vi "main.vi"() -> ()   [LabVIEW 2023]
uses:
  <vilib>/vision/Image Controls.llb/IMAQ Image.ctl
  <vilib>/vision/Shape Detection.llb/ShapeDetectionMatchOptions.ctl
  <vilib>/vision/Pattern Matching.llb/IMAQ Match Range Setting.ctl
  <vilib>/vision/NI_Vision_Development_Module.lvlib
panel:
  out "Triangles":i32
  out "String":string
  out "Rectangles":i32
  out "Circles":i32
  out "Obraz":T1(plugin-control)
  in  "Output Path":path
  in  "Input Path":path=path "C:/Users/kacpe/Desktop/OSP/testp.png"
  in  "Refresh Button":bool
  in  "Process Stop Button":bool
  in  "Save As Button":bool
  in  "Open Button":bool
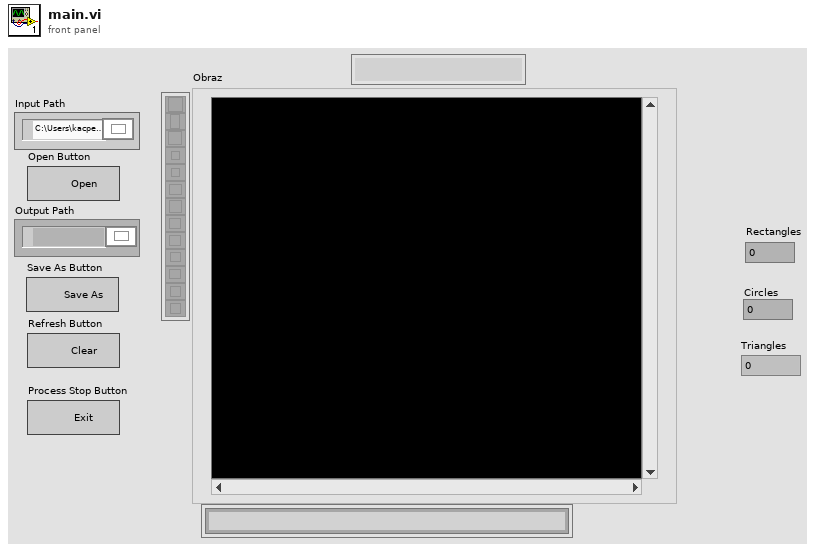
[diagram p1: front panel]
types:
  T1 = typedef "IMAQ Image.ctl" = refnum<image>
  T2 = enum32{"Invalid", "Standard", "Closed", "Hidden", "Minimized", "Maximized"}
  T3 = enum32{"invalid app kind", "Development System", "Run Time System", "Student Edition", "Embedded LabVIEW", "Evaluation", "Custom"}
  T4 = cluster{"Position":cluster{"x":sgl, "y":sgl}, "Angle":sgl, "Scale":sgl, "Score":sgl, "Bounding Box":cluster{"x":sgl, "y":sgl}[]}[]
  T5 = cluster{"Corners":cluster{"X":sgl, "Y":sgl}[], "Angle":dbl, "Width":dbl, "Height":dbl, "Score":dbl}[]
  T6 = cluster{"Position":cluster{"X":sgl, "Y":sgl}, "Radius":dbl, "Score":dbl}[]
  T7 = cluster{"Left":i32, "Top":i32, "Right":i32, "Bottom":i32}
  T8 = cluster{"Min Width":dbl, "Max Width":dbl, "Min Height":dbl, "Max Height":dbl}
  T9 = cluster{"Core":cluster{"Current VI Reference":refnum<vi>, "Close Panel on Exit?":bool}, "Obraz":T1, enum16{"null", "kwadrat", "kolo", "trojkat"}, "Rectangles 2":cluster{"Corners":cluster{"X":sgl, "Y":sgl}[], "Angle":dbl, "Width":dbl, "Height":dbl, "Score":dbl}[], "Circles":cluster{"Position":cluster{"X":sgl, "Y":sgl}, "Radius":dbl, "Score":dbl}[], "Matches (pixel)":cluster{"Position":cluster{"x":sgl, "y":sgl}, "Angle":sgl, "Scale":sgl, "Score":sgl, "Bounding Box":cluster{"x":sgl, "y":sgl}[]}[], "Znak":string}
  T10 = cluster{"Current VI Reference":refnum<vi>, "Close Panel on Exit?":bool}
  T11 = cluster{"Position":cluster{"x":sgl, "y":sgl}, "Angle":sgl, "Scale":sgl, "Score":sgl, "Bounding Box":cluster{"x":sgl, "y":sgl}[]}
  T12 = typedef "ShapeDetectionMatchOptions.ctl" = cluster{"Rotation":bool, "Scale":bool, "Occlusion":bool, "Range Settings":T13[]}
  T13 = typedef "IMAQ Match Range Setting.ctl" = cluster{"Match Constraints":u32, "Min":dbl, "Max":dbl}
  T14 = typedef "Image Type" = u32
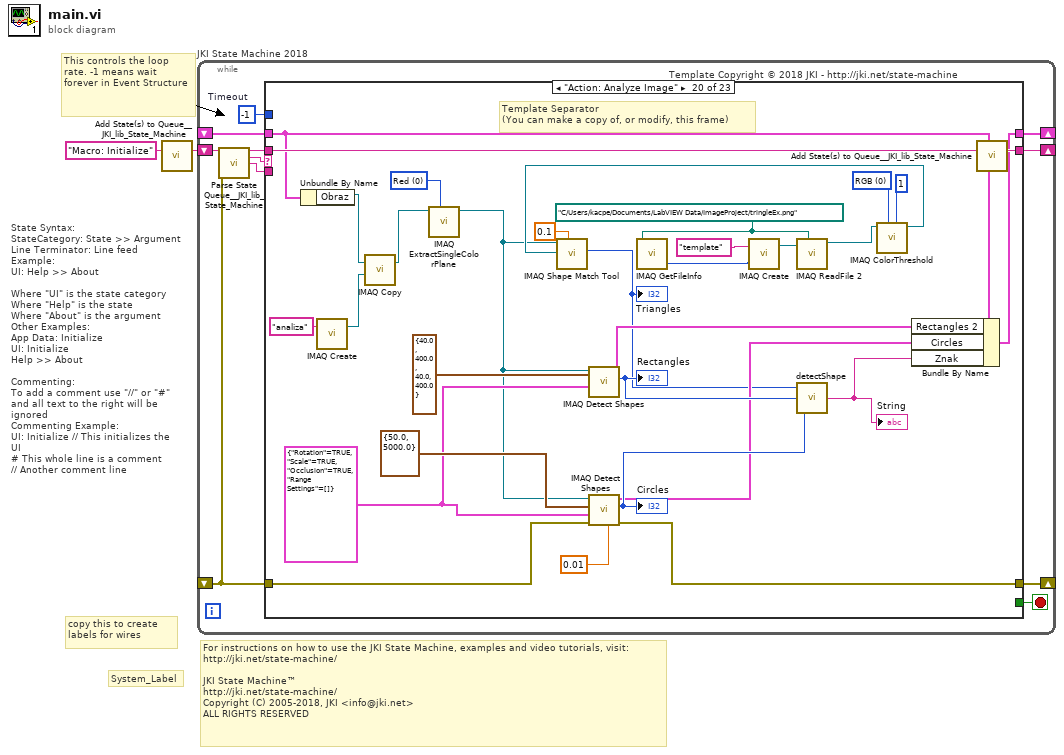
[diagram p0: block diagram]
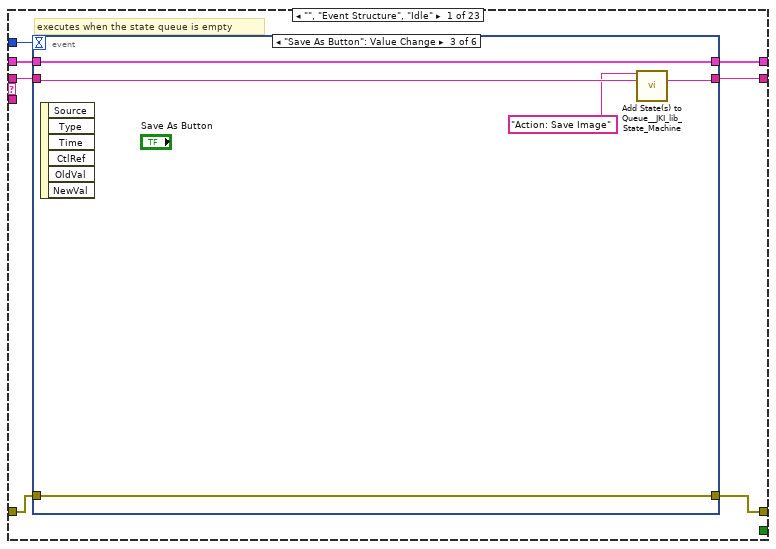
[diagram p2: hidden frame]
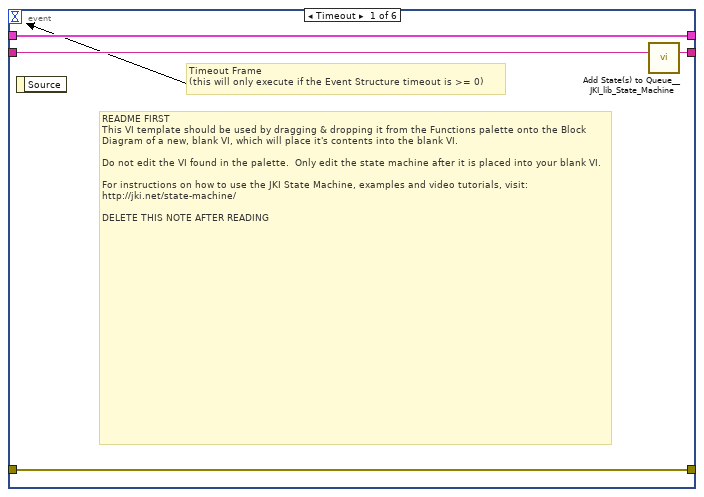
[diagram p3: hidden frame]
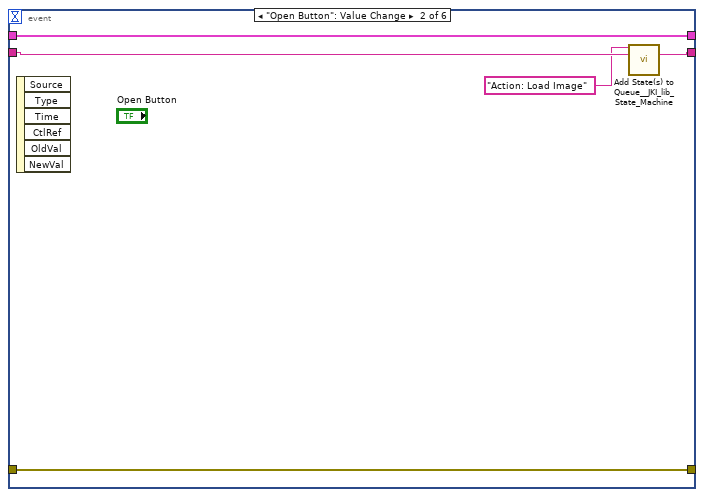
[diagram p4: hidden frame]
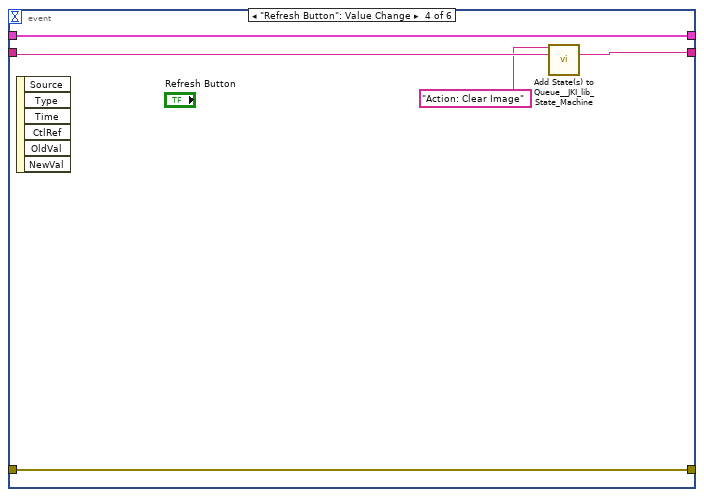
[diagram p5: hidden frame]
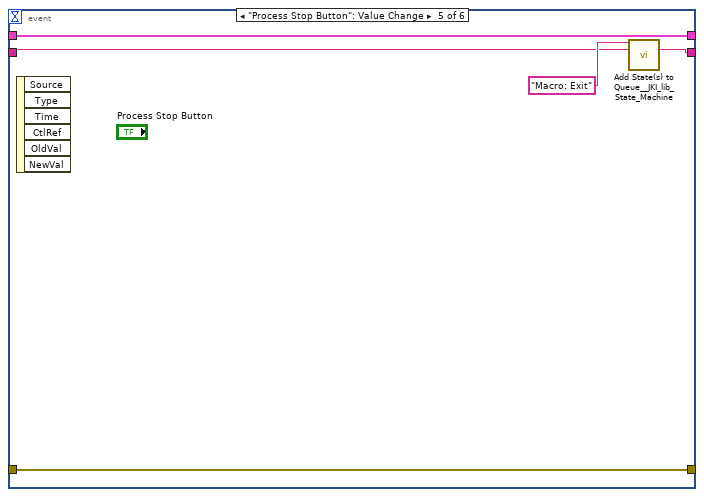
[diagram p6: hidden frame]
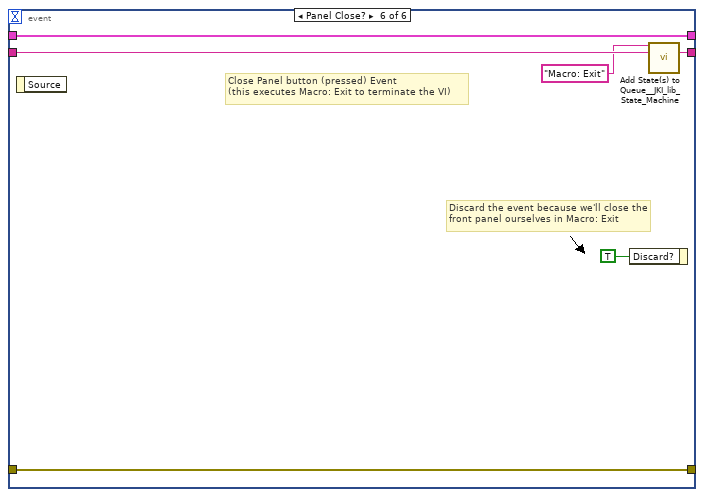
[diagram p7: hidden frame]
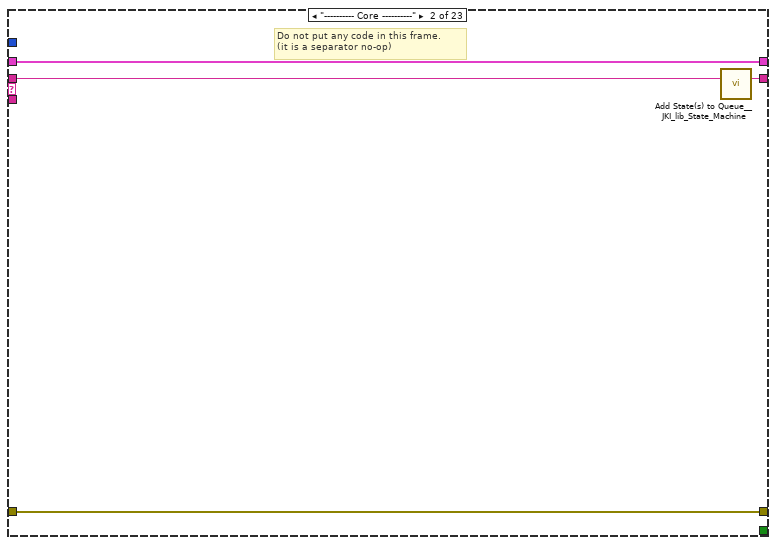
[diagram p8: hidden frame]
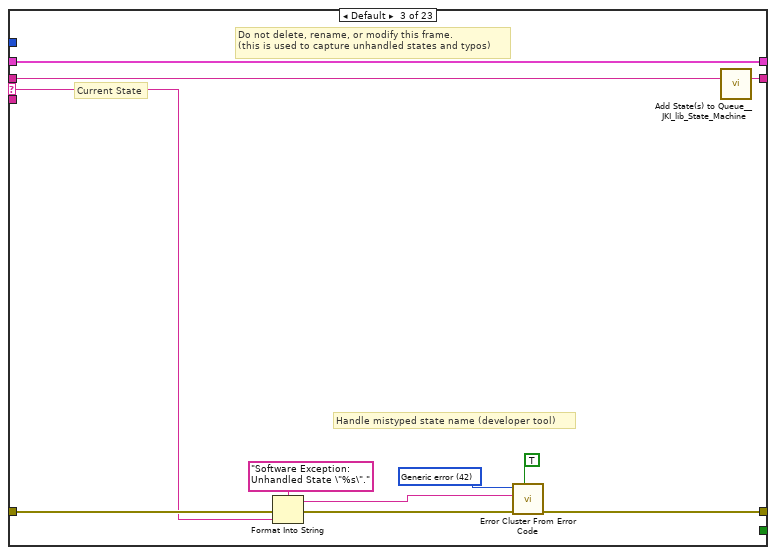
[diagram p9: hidden frame]
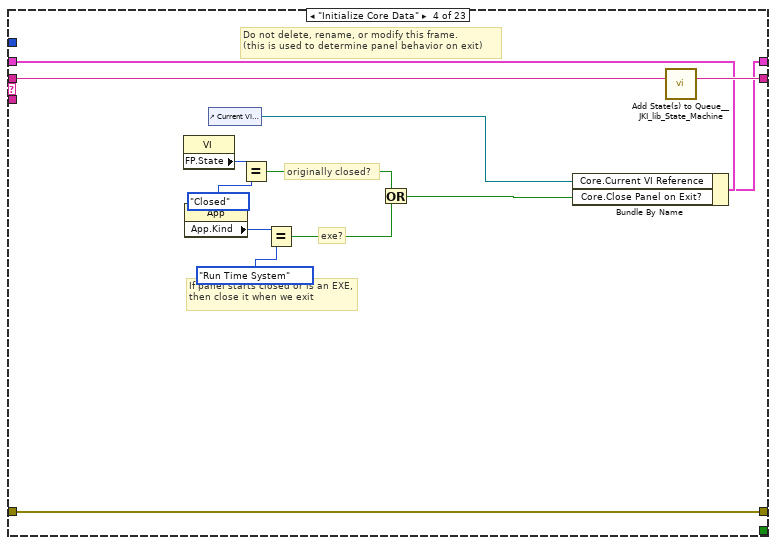
[diagram p10: hidden frame]
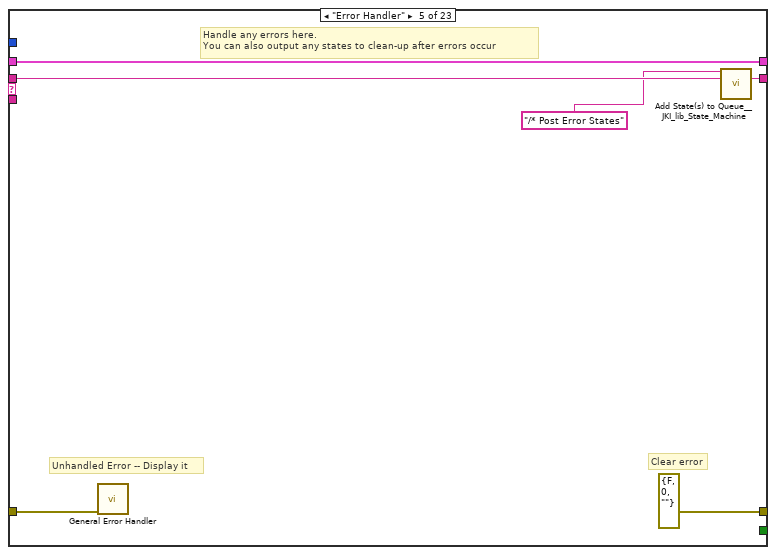
[diagram p11: hidden frame]
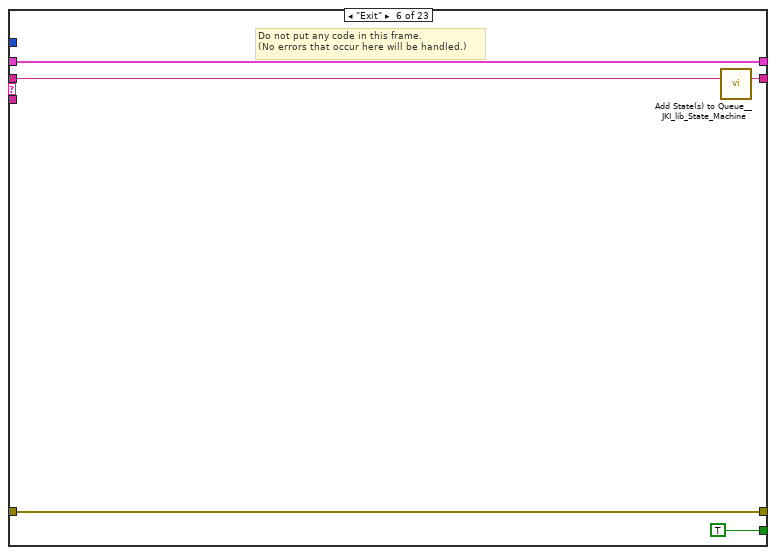
[diagram p12: hidden frame]
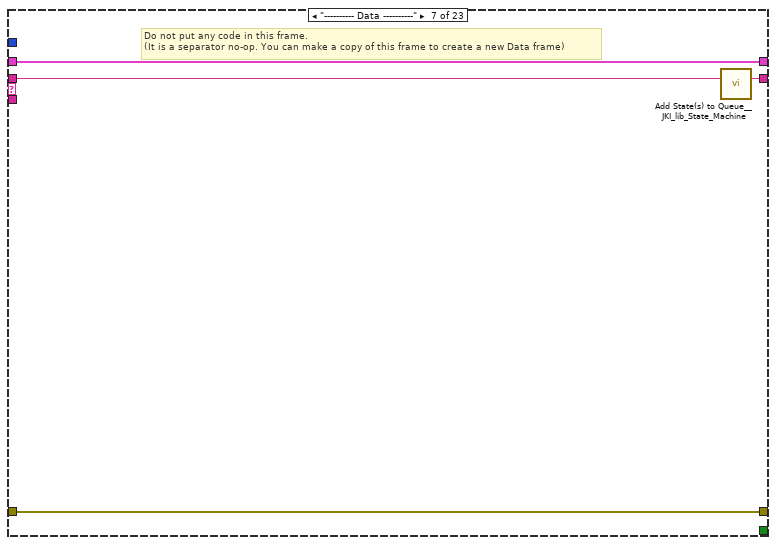
[diagram p13: hidden frame]
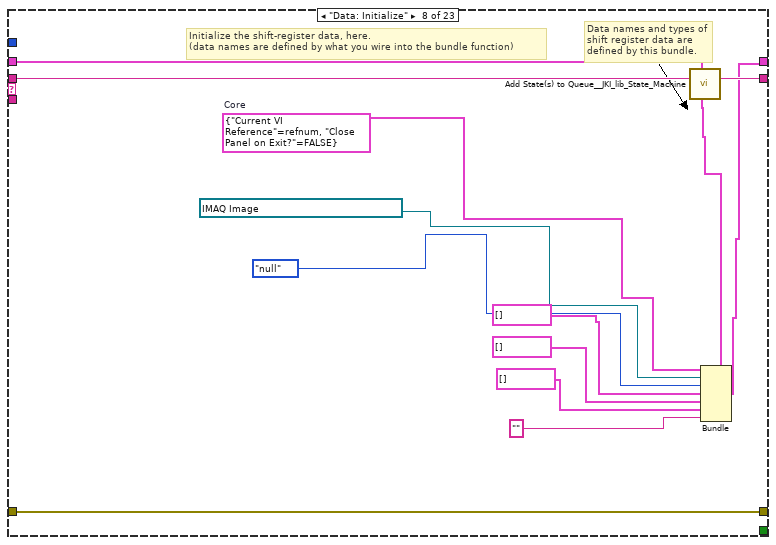
[diagram p14: hidden frame]
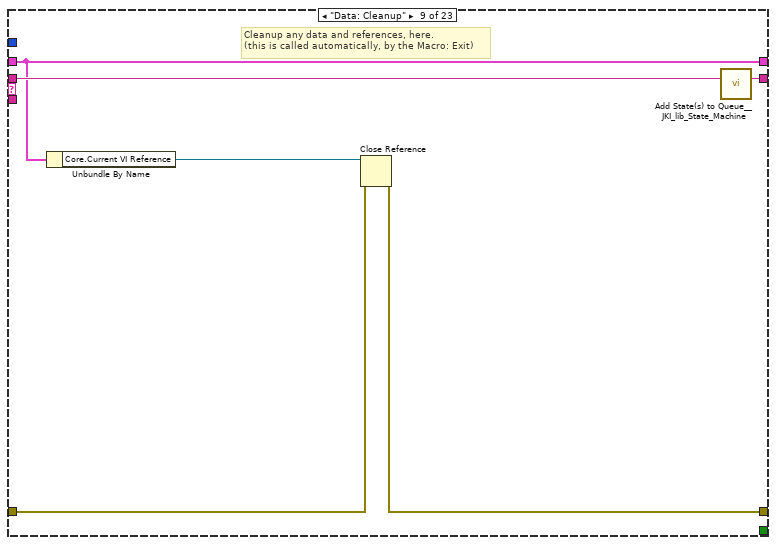
[diagram p15: hidden frame]
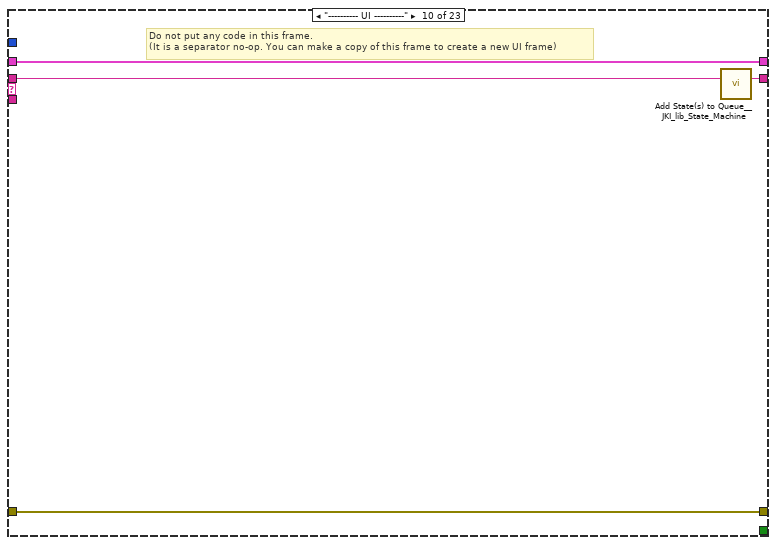
[diagram p16: hidden frame]
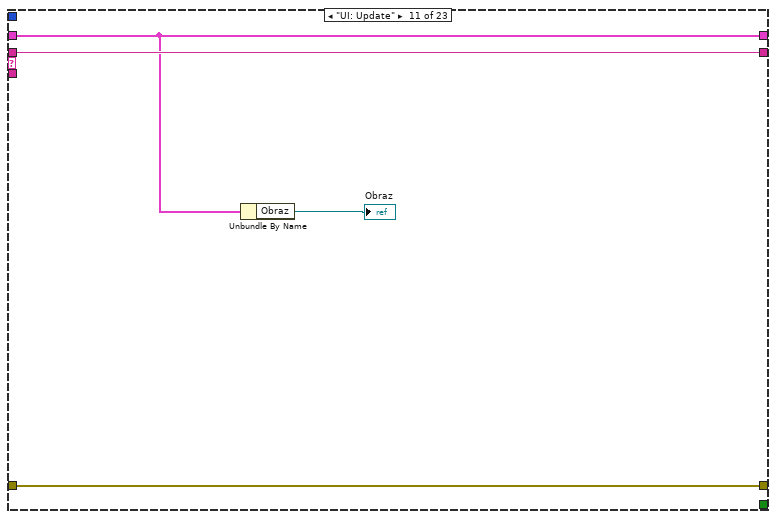
[diagram p17: hidden frame]
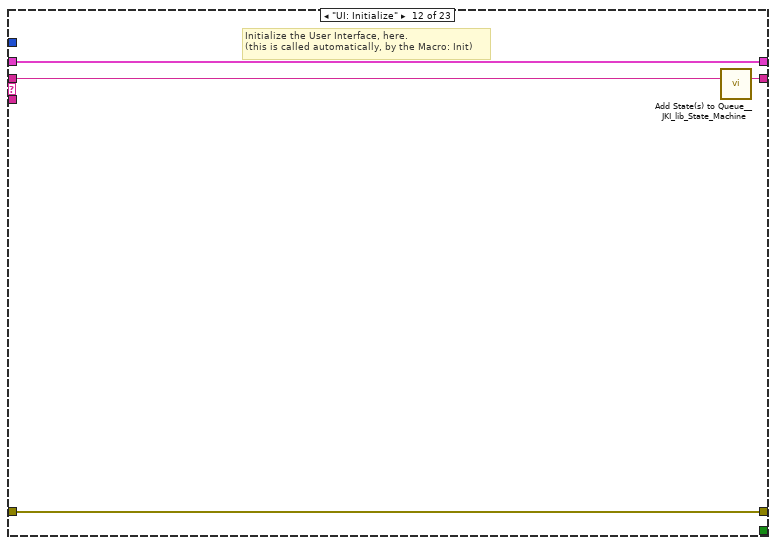
[diagram p18: hidden frame]
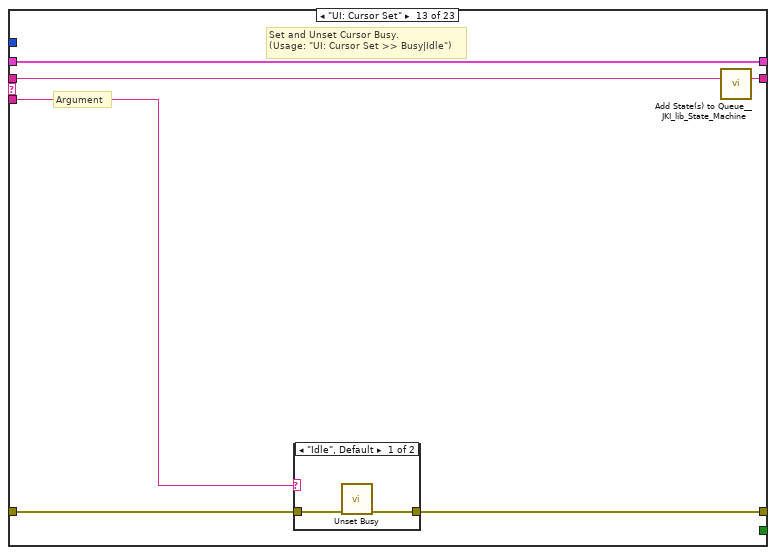
[diagram p19: hidden frame]
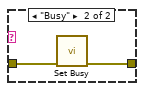
[diagram p20: hidden frame]
diagram:
  # "For instructions on how to use the JKI State Machine, examples and video tutorials, visit:\nhttp://jki.net/state-machine/\n\nJKI State Machine™\nhttp://jki.net/state-machine/\nCopyright (C) 2005-2018, JKI <info@jki.net>\nALL RIGHTS RESERVED"
  # "State Syntax:\nStateCategory: State >> Argument\nLine Terminator: Line feed\nExample:\nUI: Help >> About\n\nWhere \"UI\" is the state category\nWhere \"Help\" is the state\nWhere \"About\" is the argument\nOther Examples:\nApp Data: Initialize\nUI: Initialize\nHelp >> About\n\nCommenting:\nTo add a comment use \"//\" or \"#\" and all text to the right will be ignored\nCommenting Example:\nUI: Initialize // This initializes the UI\n# This whole line is a comment\n// Another comment line"
  # "copy this to create labels for wires"
  # "This controls the loop rate. -1 means wait forever in Event Structure"
  # "System_Label"
  n1 = call <vilib>:"Add State(s) to Queue__JKI_lib_State_Machine.vi"("State(s) in (\"\")"="Macro: Initialize") -> ("States Out"=w2:string)  [unwired: 14 in]
  n2 = while "JKI State Machine 2018" {
    shift-right: [w6] -> _
    shift-left: _ -> [w5]
    shift-right: [w9] -> _
    shift-left: _ -> [w3]
    shift-right: [w8] -> _
    shift-left: w2 -> [w10]
    stop <- w7 stop-if-true
    w4 = -1  # Timeout
    # "Template Copyright © 2018 JKI - http://jki.net/state-machine"
    n3 = call <vilib>:"Parse State Queue__JKI_lib_State_Machine.vi"("State Queue"=w10, "Error In (no error)"=w3) -> ("Remaining States"=w12:string, "Current State"=w13:string, "Arguments"=w11:string)  [unwired: 11 in]
    n4 = case shown="\"Action: Analyze Image\"" w13 {
      selector: w13 -> [_ _ w55 _ _ _ _ _ _ _ _ _ _ _ _ _ _ _ _ _ _ _ _]
      tunnel: w12 -> [w20 w54 w59 w78 w84 w89 w93 w105 w111 w115 w118 w123 w129 w140 w204 w209 w219 w223 w237 w288 w299 w306 w313]
      tunnel: w11 -> [_ _ _ _ _ _ _ _ _ _ _ _ w124 w135 _ _ _ _ _ _ _ _ _]
      tunnel: w5 -> [w18 w51 w57 w67 w81 w87 w90 w95 w107 w112 w117 w121 w127 w134 w201 w206 w211 w220 w229 w266 w290 w301 w308]
      tunnel: [w17 w52 w61 w76 errorcluster {"status"=FALSE, "code"=0, "source"=""} ("error out") w86 w91 w103 w108 w113 w119 w120 w125 w137 w202 w207 w217 w221 w234 w286 w293 w304 w311] -> w9
      tunnel: w3 -> [w16 w52 w60 w76 w80 w86 w91 w103 w109 w113 w119 w120 w126 w138 w202 w207 w217 w221 w233 w285 w293 w303 w311]
      tunnel: [w19 w53 w58 w77 w83 w88 w92 w104 w110 w114 w118 w122 w128 w139 w203 w208 w218 w222 w236 w287 w298 w305 w312] -> w8
      tunnel: [_ _ _ _ _ TRUE _ _ _ _ _ _ _ _ _ _ _ _ _ _ _ _ _] -> w7
      tunnel: [w15 w51 w57 w66 w81 w87 w90 w94 w107 w112 w117 w121 w127 w134 w201 w206 w211 w220 w230 w267 w291 w301 w309] -> w6
      tunnel: w4 -> [w14 _ _ _ _ _ _ _ _ _ _ _ _ _ _ _ _ _ _ _ _ _ _]
      frame "", "Event Structure", "Idle" {
        # "executes when the state queue is empty"
        n5 = event shown="[2] \"Save As Button\": Value Change" {
          selector: _ -> [_ _ _ _ _ _]
          dyn-events: _ -> [_ _ _ _ _ _]
          timeout: w14 -> [_ _ _ _ _ _]
          tunnel: w20 -> [w24 w27 w31 w36 w41 w50]
          tunnel: [w23 w28 w32 w37 w43 w49] -> w19
          tunnel: w18 -> [w21 w29 w34 w39 w44 w47]
          tunnel: [w22 w25 w33 w38 w40 w48] -> w17
          tunnel: w16 -> [w22 w25 w33 w38 w40 w48]
          tunnel: [w21 w29 w34 w39 w44 w47] -> w15
          event Timeout {
            # "README FIRST\nThis VI template should be used by dragging & dropping it from the Functions palette onto the Block Diagram of a new, blank VI, which will place it's contents into the blank VI.\n\nDo not edit the VI found in the palette.  Only edit the state machine after it is placed into your blank VI.\n\nFor instructions on how to use the JKI State Machine, examples and video tutorials, visit:\nhttp://jki.net/state-machine/\n\nDELETE THIS NOTE AFTER READING"
            # "Timeout Frame\n(this will only execute if the Event Structure timeout is >= 0)"
            n6 = event-data() -> ()  [unwired: 1 in, 1 out]
            n7 = call <vilib>:"Add State(s) to Queue__JKI_lib_State_Machine.vi"("State(s) in (\"\")"=w24) -> ("States Out"=w23:string)  [unwired: 14 in]
          }
          event "Open Button": Value Change {
            n8 = event-data() -> ()  [unwired: 1 in, 6 out]
            n9 = call <vilib>:"Add State(s) to Queue__JKI_lib_State_Machine.vi"("State(s) in Front (\"\")"="Action: Load Image" ("State(s) in Front (\"\")"), "State(s) in (\"\")"=w27) -> ("States Out"=w28:string)  [unwired: 13 in]
          }
          event "Save As Button": Value Change {
            n10 = event-data() -> ()  [unwired: 1 in, 6 out]
            n11 = call <vilib>:"Add State(s) to Queue__JKI_lib_State_Machine.vi"("State(s) in Front (\"\")"="Action: Save Image" ("State(s) in Front (\"\")"), "State(s) in (\"\")"=w31) -> ("States Out"=w32:string)  [unwired: 13 in]
          }
          event "Refresh Button": Value Change {
            n12 = event-data() -> ()  [unwired: 1 in, 6 out]
            n13 = call <vilib>:"Add State(s) to Queue__JKI_lib_State_Machine.vi"("State(s) in Front (\"\")"="Action: Clear Image" ("State(s) in Front (\"\")"), "State(s) in (\"\")"=w36) -> ("States Out"=w37:string)  [unwired: 13 in]
          }
          event "Process Stop Button": Value Change {
            n14 = event-data() -> ()  [unwired: 1 in, 6 out]
            n15 = call <vilib>:"Add State(s) to Queue__JKI_lib_State_Machine.vi"("State(s) in Front (\"\")"="Macro: Exit", "State(s) in (\"\")"=w41) -> ("States Out"=w43:string)  [unwired: 13 in]
          }
          event Panel Close? {
            # "Discard the event because we'll close the front panel ourselves in Macro: Exit"
            # "Close Panel button (pressed) Event\n(this executes Macro: Exit to terminate the VI)"
            n16 = event-data() -> ()  [unwired: 1 in, 1 out]
            n17 = event-data("Discard?"=TRUE) -> ()  [unwired: 1 in, 1 out]
            n18 = call <vilib>:"Add State(s) to Queue__JKI_lib_State_Machine.vi"("State(s) in Front (\"\")"="Macro: Exit", "State(s) in (\"\")"=w50) -> ("States Out"=w49:string)  [unwired: 13 in]
          }
        }
      }
      frame "---------- Core ----------" {
        # "Do not put any code in this frame.\n(it is a separator no-op)"
        n19 = call <vilib>:"Add State(s) to Queue__JKI_lib_State_Machine.vi"("State(s) in (\"\")"=w54) -> ("States Out"=w53:string)  [unwired: 14 in]
      }
      frame Default {
        w64 = 42 items=["No error", "Argument error", "Memory is full", "Out of zone", "End of file", "File already open", "Generic file I/O error", "File not found", "File permission error", "Disk is full", "Duplicate path", "Too many files open", "System feature not enabled", "Resource file not found", "Cannot add resource", "Resource not found", "Image not found", "Image memory error", "Pen does not exist", "Config type invalid", "Config token not found", "Config parse error", "Config memory error", "Bad external code format", "Bad external code offset", "External code not present", "Null window", "Destroy window error", "Null menu", "Print aborted", "Bad print record", "Print driver error", "Windows error during printing", "Memory error during printing", "Print dialog error", "Generic print error", "Invalid device refnum", "Device not found", "Device parameter error", "Device unit error", "Cannot open device", "Device call aborted", "Generic error", "Cancelled by user", "Object ID too low", "Object ID too high", "Object not in heap", "Unknown heap", "Unknown object (invalid DefProc)", "Unknown object (DefProc not in table)", "Message out of range", "Invalid (null) method", "Unknown message", "Manager call not supported", "Bad address", "Network operation in progress", "Network operation timed out", "Connection is busy", "Network attribute not supported", "Network error", "Address in use", "System out of memory", "Connection aborted", "Connection refused", "Not connected", "Already connected", "Connection closed", "Initialization error (interapplication manager)", "Bad occurrence", "Wait on unbound occurrence handler", "Occurrence queue overflow", "Datalog type conflict", "Unused", "Unrecognized type (interapplication manager)", "Memory corrupt", "Failed to make temporary DLL", "Old CIN version", "Drag socket not found", "Failed to load drop-object", "Failed to register OLE object", "Failed to release OLE object", "Format specifier type mismatch", "Unknown format specifier", "Too few format specifiers", "Too many format specifiers", "Scan failed", "Newer CIN version", "Error converting to variant", "Runtime menu error", "Password tampered", "Variant attribute not found", "Incompatible variant data type", "Event data is not available", "Event Store is not present", "Occurrence is not found", "Event Queue is not created", "Event info is not available", "Refnum passed is NULL", "Error retrieving Class GUID", "Error retrieving CoClass GUID", "Error retrieving TypeLib GUID.", "Bad built application magic bytes.", "Specific driver is different from the specific driver associated with the Logical Name.", "There is no session opened to the class driver.", "Max Error", "MAX - Error with config objects", "MAX - Error loading configuration", "MAX - Group not supported"]
        # "Current State"
        # "Do not delete, rename, or modify this frame.\n(this is used to capture unhandled states and typos)"
        # "Handle mistyped state name (developer tool)"
        n20 = Format Into String(format string="Software Exception: Unhandled State \"%s\"." ("message"), error in=w60, w55) -> (resulting string=w63:string, error out=w62:errorcluster)  [unwired: 1 in]
        n21 = call <vilib>:"Error Cluster From Error Code.vi"("show call chain? (False)"=TRUE, "error in (no error)"=w62, "error message (\"\")"=w63, "error code (0)"=w64) -> ("error out"=w61:errorcluster)  [unwired: 5 in]
        n22 = call <vilib>:"Add State(s) to Queue__JKI_lib_State_Machine.vi"("State(s) in (\"\")"=w59) -> ("States Out"=w58:string)  [unwired: 14 in]
      }
      frame "Initialize Core Data" {
        # "Do not delete, rename, or modify this frame.\n(this is used to determine panel behavior on exit)"
        # "originally closed?"
        # "exe?"
        # "If panel starts closed or is an EXE, then close it when we exit"
        n23 = property class="VI"() -> ("FP.State"=w70:T2)  [unwired: 2 in, 2 out]
        n24 = property class="App"() -> ("App.Kind"=w75:T3)  [unwired: 2 in, 2 out]
        n25 = control-ref of="Current VI Reference"() -> (w71:refnum<vi>)
        n26 = Equal?(x=w70, y=T2."Closed" ("Front Panel Window:State")) -> (x = y?=w68:bool)
        n27 = Equal?(x=w75, y=T3."Run Time System" ("Application:Kind")) -> (x = y?=w73:bool)
        n28 = Or(x=w68, y=w73) -> (x .or. y?=w72:bool)
        n29 = Bundle By Name(cluster=w67, "Core.Current VI Reference"=w71, "Core.Close Panel on Exit?"=w72) -> (w66:T9)
        n30 = call <vilib>:"Add State(s) to Queue__JKI_lib_State_Machine.vi"("State(s) in (\"\")"=w78) -> ("States Out"=w77:string)  [unwired: 14 in]
      }
      frame "Error Handler" {
        # "Unhandled Error -- Display it"
        # "Handle any errors here.\nYou can also output any states to clean-up after errors occur"
        # "Clear error"
        n31 = call <vilib>:"General Error Handler.vi"("error in (no error)"=w80) -> ()  [unwired: 10 in, 5 out]
        n32 = call <vilib>:"Add State(s) to Queue__JKI_lib_State_Machine.vi"("State(s) in Front (\"\")"="/* Post Error States", "State(s) in (\"\")"=w84) -> ("States Out"=w83:string)  [unwired: 13 in]
      }
      frame "Exit" {
        # "Do not put any code in this frame.\n(No errors that occur here will be handled.)"
        n33 = call <vilib>:"Add State(s) to Queue__JKI_lib_State_Machine.vi"("State(s) in (\"\")"=w89) -> ("States Out"=w88:string)  [unwired: 14 in]
      }
      frame "---------- Data ----------" {
        # "Do not put any code in this frame.\n(It is a separator no-op. You can make a copy of this frame to create a new Data frame)"
        n34 = call <vilib>:"Add State(s) to Queue__JKI_lib_State_Machine.vi"("State(s) in (\"\")"=w93) -> ("States Out"=w92:string)  [unwired: 14 in]
      }
      frame "Data: Initialize" {
        w96 = T10 {"Current VI Reference"=refnum, "Close Panel on Exit?"=FALSE}  # Core
        # "Data names and types of shift register data are defined by this bundle."
        # "Initialize the shift-register data, here.\n(data names are defined by what you wire into the bundle function)"
        n35 = call <vilib>:"Add State(s) to Queue__JKI_lib_State_Machine.vi"("State(s) in (\"\")"=w105) -> ("States Out"=w104:string)  [unwired: 14 in]
        n36 = Bundle(cluster=w95, "Core"=w96, "Obraz"=T1 refnum, enum16{"null", "kwadrat", "kolo", "trojkat"}."null", "Rectangles 2"=T5 [], "Circles"=T6 [], "Matches (pixel)"=T4 [], "Znak"="") -> (w94:T9)
      }
      frame "Data: Cleanup" {
        # "Cleanup any data and references, here.\n(this is called automatically, by the Macro: Exit)"
        n37 = Unbundle By Name(w107) -> ("Core.Current VI Reference"=w106:refnum<vi>)
        n38 = Close Reference(reference=w106, error in (no error)=w109) -> (error out=w108:errorcluster)
        n39 = call <vilib>:"Add State(s) to Queue__JKI_lib_State_Machine.vi"("State(s) in (\"\")"=w111) -> ("States Out"=w110:string)  [unwired: 14 in]
      }
      frame "---------- UI ----------" {
        # "Do not put any code in this frame.\n(It is a separator no-op. You can make a copy of this frame to create a new UI frame)"
        n40 = call <vilib>:"Add State(s) to Queue__JKI_lib_State_Machine.vi"("State(s) in (\"\")"=w115) -> ("States Out"=w114:string)  [unwired: 14 in]
      }
      frame "UI: Update" {
        n41 = Unbundle By Name(w117) -> ("Obraz"=→"Obraz":T1)
      }
      frame "UI: Initialize" {
        # "Initialize the User Interface, here.\n(this is called automatically, by the Macro: Init)"
        n42 = call <vilib>:"Add State(s) to Queue__JKI_lib_State_Machine.vi"("State(s) in (\"\")"=w123) -> ("States Out"=w122:string)  [unwired: 14 in]
      }
      frame "UI: Cursor Set" {
        # "Argument"
        # "Set and Unset Cursor Busy.\n(Usage: \"UI: Cursor Set >> Busy|Idle\")"
        n43 = case shown="\"Idle\", Default" w124 {
          tunnel: w126 -> [w131 w133]
          tunnel: [w130 w132] -> w125
          frame "Idle", Default {
            n44 = call <vilib>:"Unset Busy.vi"("error in (no error)"=w131) -> ("error out"=w130:errorcluster)  [unwired: 10 in]
          }
          frame "Busy" {
            n45 = call <vilib>:"Set Busy.vi"("error in (no error)"=w133) -> ("error out"=w132:errorcluster)  [unwired: 9 in, 1 out]
          }
        }
        n46 = call <vilib>:"Add State(s) to Queue__JKI_lib_State_Machine.vi"("State(s) in (\"\")"=w129) -> ("States Out"=w128:string)  [unwired: 14 in]
      }
      frame "UI: Front Panel State" {
        # "Argument"
        # "Set Front Panel Open or Closed\n(Usage: \"UI: Front Panel State >> Open|Close\")"
        n47 = Unbundle By Name(w134) -> ("Core.Current VI Reference"=w136:refnum<vi>)
        n48 = case shown="\"Minimize\", \"Minimized\"" w135 {
          tunnel: w138 -> [w146 w159 w170 w182 w194]
          tunnel: [w147 w160 w171 w183 w195] -> w137
          tunnel: w136 -> [_ _ _ _ _]
          frame "Open", "Standard", Default {
            w141 = T2."Standard" ("State")
            n49 = property class="VI"(error in=w146) -> (reference out=w144:refnum<vi>, error out=w145:errorcluster, "FP.State"=w143:T2)  [unwired: 1 in]
            n50 = Not Equal?(x=w143, y=w141) -> (x != y?=w142:bool)
            n51 = case shown="True" w142 {
              tunnel: [w151 w153] -> w147
              tunnel: w145 -> [w150 w153]
              tunnel: w144 -> [w149 _]
              tunnel: w141 -> [w148 _]
              frame True {
                n52 = invoke class="VI" method="FP.Open"(reference=w149, error in=w150, "Activate"=TRUE, "State"=w148) -> (error out=w151:errorcluster)  [unwired: 1 in, 4 out]
              }
              frame False {
              }
            }
          }
          frame "Close", "Closed" {
            n53 = property class="VI"(error in=w159) -> (reference out=w157:refnum<vi>, error out=w158:errorcluster, "FP.State"=w155:T2)  [unwired: 1 in]
            n54 = Not Equal?(x=w155, y=T2."Closed" ("Front Panel Window:State")) -> (x != y?=w154:bool)
            n55 = case shown="True" w154 {
              tunnel: [w161 w164] -> w160
              tunnel: w158 -> [w161 w163]
              tunnel: w157 -> [_ w162]
              frame False {
              }
              frame True {
                n56 = invoke class="VI" method="FP.Close"(reference=w162, error in=w163) -> (error out=w164:errorcluster)  [unwired: 1 in, 2 out]
              }
            }
          }
          frame "Hidden", "Hide" {
            w165 = T2."Hidden" ("State")
            n57 = property class="VI"(error in=w170) -> (reference out=w168:refnum<vi>, error out=w169:errorcluster, "FP.State"=w167:T2)  [unwired: 1 in]
            n58 = Not Equal?(x=w167, y=w165) -> (x != y?=w166:bool)
            n59 = case shown="True" w166 {
              tunnel: [w175 w176] -> w171
              tunnel: w169 -> [w174 w176]
              tunnel: w168 -> [w173 _]
              tunnel: w165 -> [w172 _]
              frame True {
                n60 = invoke class="VI" method="FP.Open"(reference=w173, error in=w174, "State"=w172) -> (error out=w175:errorcluster)  [unwired: 2 in, 4 out]
              }
              frame False {
              }
            }
          }
          frame "Minimize", "Minimized" {
            w177 = T2."Minimized" ("State")
            n61 = property class="VI"(error in=w182) -> (reference out=w180:refnum<vi>, error out=w181:errorcluster, "FP.State"=w179:T2)  [unwired: 1 in]
            n62 = Not Equal?(x=w179, y=w177) -> (x != y?=w178:bool)
            n63 = case shown="True" w178 {
              tunnel: [w187 w188] -> w183
              tunnel: w181 -> [w186 w188]
              tunnel: w180 -> [w185 _]
              tunnel: w177 -> [w184 _]
              frame True {
                n64 = invoke class="VI" method="FP.Open"(reference=w185, error in=w186, "State"=w184) -> (error out=w187:errorcluster)  [unwired: 2 in, 4 out]
              }
              frame False {
              }
            }
          }
          frame "Maximize", "Maximized" {
            w189 = T2."Maximized" ("State")
            n65 = property class="VI"(error in=w194) -> (reference out=w192:refnum<vi>, error out=w193:errorcluster, "FP.State"=w191:T2)  [unwired: 1 in]
            n66 = Not Equal?(x=w191, y=w189) -> (x != y?=w190:bool)
            n67 = case shown="True" w190 {
              tunnel: [w199 w200] -> w195
              tunnel: w193 -> [w198 w200]
              tunnel: w192 -> [w197 _]
              tunnel: w189 -> [w196 _]
              frame True {
                n68 = invoke class="VI" method="FP.Open"(reference=w197, error in=w198, "State"=w196) -> (error out=w199:errorcluster)  [unwired: 2 in, 4 out]
              }
              frame False {
              }
            }
          }
        }
        n69 = call <vilib>:"Add State(s) to Queue__JKI_lib_State_Machine.vi"("State(s) in (\"\")"=w140) -> ("States Out"=w139:string)  [unwired: 14 in]
      }
      frame "---------- Macro ----------" {
        # "Do not put any code in this frame.\n(It is a separator no-op. You can make a copy of this frame to create a new Macro frame)"
        n70 = call <vilib>:"Add State(s) to Queue__JKI_lib_State_Machine.vi"("State(s) in (\"\")"=w204) -> ("States Out"=w203:string)  [unwired: 14 in]
      }
      frame "Macro: Initialize" {
        w205 = "Data: Initialize\nInitialize Core Data\nUI: Initialize\nUI: Front Panel State >> Open"  # Data: Initialize Initialize Core Data UI: Initialize UI: Front Panel State >> Open
        # "Initialization Macro\n(This is called once, when the VI starts)"
        n71 = call <vilib>:"Add State(s) to Queue__JKI_lib_State_Machine.vi"("State(s) in Front (\"\")"=w205, "State(s) in (\"\")"=w209) -> ("States Out"=w208:string)  [unwired: 13 in]
      }
      frame "Macro: Exit" {
        # "Exit Macro\n(This is called once, when the VI exits)"
        n72 = Unbundle By Name(w211) -> ("Core.Close Panel on Exit?"=w210:bool)
        n73 = Select(t="UI: Front Panel State >> Close", s=w210, f="") -> (s? t:f=w214:string)
        n74 = call <vilib>:"Add State(s) to Queue__JKI_lib_State_Machine.vi"("State(s) in (\"\")"=w214, "State(s) at Back (\"\")"="Data: Cleanup\nExit") -> ("States Out"=w212:string)  [unwired: 13 in]
        n75 = call <vilib>:"Add State(s) to Queue__JKI_lib_State_Machine.vi"("State(s) in Front (\"\")"=w212, "State(s) in (\"\")"=w219) -> ("States Out"=w218:string)  [unwired: 13 in]
      }
      frame "---------- Action ----------" {
        # "Template Separator\n(You can make a copy of, or modify, this frame)"
        n76 = call <vilib>:"Add State(s) to Queue__JKI_lib_State_Machine.vi"("State(s) in (\"\")"=w223) -> ("States Out"=w222:string)  [unwired: 14 in]
      }
      frame "Action: Draw Boundling Box" {
        # "Template Separator\n(You can make a copy of, or modify, this frame)"
        n77 = Unbundle By Name(w229) -> ("Obraz"=w235:T1, "Rectangles 2"=w227:T5, "Circles"=w226:T6, "Znak"=w228:string, "Matches (pixel)"=w224:T4)
        n78 = case shown="\"Znak ostrzegawczy\"" w228 {
          tunnel: w227 -> [w239 _ _ _ _]
          tunnel: w226 -> [_ _ _ _ w257]
          tunnel: [w238 T7 {"Left"=0, "Top"=0, "Right"=0, "Bottom"=0} ("output cluster") T7 {"Left"=0, "Top"=0, "Right"=0, "Bottom"=0} ("output cluster") w246 w256] -> w225
          tunnel: w224 -> [_ _ _ w255 _]
          frame "Znak informacyjny" {
            n79 = call "rectangleBox.vi"("Rectangles 2"=w239) -> ("output cluster"=w238:T7)
          }
          frame "Nie rozpoznano znaku !" {
          }
          frame "", Default {
          }
          frame "Znak ostrzegawczy" {
            n80 = Index Array(array=w255, index #1=0 ("index"), index #2=2 ("index")) -> (element #1=w252:T11, element #2=w251:T11)
            n81 = Unbundle By Name(w251) -> ("Bounding Box"=w250:cluster{"x":sgl, "y":sgl}[])
            n82 = Unbundle By Name(w252) -> ("Position.x"=w245:sgl, "Position.y"=w244:sgl)
            n83 = Index Array(array=w250, index=0) -> (element=w248:cluster{"x":sgl, "y":sgl})
            n84 = Unbundle By Name(w248) -> ("x"=w243:sgl, "y"=w242:sgl)
            n85 = Bundle By Name(cluster=T7 {"Left"=0, "Top"=0, "Right"=0, "Bottom"=0} ("output cluster"), "Left"=w245, "Top"=w244, "Right"=w243, "Bottom"=w242) -> (w246:T7)
          }
          frame "Znak nakazu lub zakazu" {
            n86 = call "circleBox.vi"("Circles 3"=w257) -> ("output cluster"=w256:T7)
          }
        }
        n87 = call "IMAQ Overlay Rectangle"("Color"=u32 16711680, "error in (no error)"=w233, "Rectangle"=w225, "Image"=w235) -> ("error out"=w234:errorcluster, "Image Out"=w231:T1)  [unwired: 6 in]
        n88 = Bundle By Name(cluster=w229, "Obraz"=w231) -> (w230:T9)
        n89 = call <vilib>:"Add State(s) to Queue__JKI_lib_State_Machine.vi"("State(s) in (\"\")"=w237) -> ("States Out"=w236:string)  [unwired: 14 in]
      }
      frame "Action: Analyze Image" {
        w264 = u16 0 items=["RGB", "HSL", "HSV", "HSI"] ("Color Mode")
        w272 = 0 items=["Red", "Green", "Blue", "Hue", "Saturation", "Luminance", "Value", "Intensity"] ("Color Plane")
        w275 = T12 {"Rotation"=TRUE, "Scale"=TRUE, "Occlusion"=TRUE, "Range Settings"=[]} ("Match Options")
        w280 = path "C:/Users/kacpe/Documents/LabVIEW Data/ImageProject/tringleEx.png" ("File Path")
        # "Template Separator\n(You can make a copy of, or modify, this frame)"
        n90 = Unbundle By Name(w266) -> ("Obraz"=w279:T1)
        n91 = call "IMAQ Create"("Image Name"="analiza") -> ("New Image"=w278:T1)  [unwired: 4 in, 1 out]
        n92 = call "IMAQ Copy"("Image Dst"=w278, "Image Src"=w279) -> ("Image Dst Out"=w273:T1)  [unwired: 4 in, 1 out]
        n93 = call "IMAQ ExtractSingleColorPlane"("Color Plane"=w272, "Image Src"=w273) -> ("Image Dst Out"=w260:T1)  [unwired: 8 in, 1 out]
        n94 = call-poly "IMAQ Detect Shapes"("Match Options"=w275, "Rectangle Descriptor"=T8 {"Min Width"=40.0, "Max Width"=400.0, "Min Height"=40.0, "Max Height"=400.0}, "Image"=w260) -> ("Number of Matches Returned"=w271:i32, "Rectangles"=w269:T5)  [unwired: 6 in, 1 out]
        "Rectangles" <- w271
        n95 = call-poly "IMAQ Detect Shapes"("Minimum match score"=0.01, "error in (no error)"=w285, "Match Options"=w275, "Circle Descriptor"=cluster{"Min Radius":dbl, "Max Radius":dbl} {"Min Radius"=50.0, "Max Radius"=5000.0}, "Image"=w260) -> ("error out"=w286:errorcluster, "Number of Matches Returned"=w270:i32, "Circles"=w268:T6)  [unwired: 4 in]
        "Circles" <- w270
        n96 = call "IMAQ GetFileInfo"("File Path"=w280) -> ("Image Type"=w282:T14)  [unwired: 4 in, 6 out]
        n97 = call "IMAQ Create"("Image Name"="template", "Image Type"=w282) -> ("New Image"=w281:T1)  [unwired: 3 in, 1 out]
        n98 = call "IMAQ ReadFile 2"("File Path"=w280, "Image"=w281) -> ("Image Out"=w262:T1)  [unwired: 5 in, 4 out]
        n99 = call "IMAQ ColorThreshold"("Replace Value"=1, "Color Mode"=w264, "Image Src"=w262) -> ("Image Dst Out"=w261:T1)  [unwired: 7 in, 1 out]
        n100 = call "IMAQ Shape Match Tool"("Tolerance"=0.1, "Image Template"=w261, "Image Src"=w260) -> ("Number of Matches"=w259:i32)  [unwired: 5 in, 3 out]
        "Triangles" <- w259
        n101 = call "detectShape.vi"("circle"=w270, "rectangle"=w271, "triangle"=w259) -> ("String"=w258:string)
        "String" <- w258
        n102 = Bundle By Name(cluster=w266, "Rectangles 2"=w269, "Circles"=w268, "Znak"=w258) -> (w267:T9)
        n103 = call <vilib>:"Add State(s) to Queue__JKI_lib_State_Machine.vi"("State(s) in (\"\")"=w288) -> ("States Out"=w287:string)  [unwired: 14 in]
      }
      frame "Action: Load Image" {
        # "Your code here.\n(You can make a copy of, or modify, this frame)"
        n104 = call "IMAQ GetFileInfo"("File Path"="Input Path") -> ("Image Type"=w295:T14)  [unwired: 4 in, 6 out]
        n105 = call "IMAQ Create"("Image Name"="image", "Image Type"=w295) -> ("New Image"=w294:T1)  [unwired: 3 in, 1 out]
        n106 = call "IMAQ ReadFile 2"("File Path"="Input Path", "Image"=w294) -> ("Image Out"=w292:T1)  [unwired: 5 in, 4 out]
        n107 = Bundle By Name(cluster=w290, "Obraz"=w292) -> (w291:T9)
        n108 = call <vilib>:"Add State(s) to Queue__JKI_lib_State_Machine.vi"("State(s) in Front (\"\")"="UI: Update\n Action: Draw Boundling Box\nAction: Analyze Image" ("State(s) in Front (\"\")"), "State(s) in (\"\")"=w299) -> ("States Out"=w298:string)  [unwired: 13 in]
      }
      frame "Action: Save Image" {
        # "Your code here.\n(You can make a copy of, or modify, this frame)"
        n109 = Unbundle By Name(w301) -> ("Obraz"=w300:T1)
        n110 = call-poly "IMAQ Write File 2"("error in (no error)"=w303, "File Path"="Output Path", "Image"=w300) -> ("error out"=w304:errorcluster)  [unwired: 7 in, 1 out]
        n111 = call <vilib>:"Add State(s) to Queue__JKI_lib_State_Machine.vi"("State(s) in (\"\")"=w306) -> ("States Out"=w305:string)  [unwired: 14 in]
      }
      frame "Action: Clear Image" {
        # "Your code here.\n(You can make a copy of, or modify, this frame)"
        n112 = Bundle By Name(cluster=w308, "Obraz"=T1 refnum) -> (w309:T9)
        n113 = call <vilib>:"Add State(s) to Queue__JKI_lib_State_Machine.vi"("State(s) in Front (\"\")"="UI: Update" ("State(s) in Front (\"\")"), "State(s) in (\"\")"=w313) -> ("States Out"=w312:string)  [unwired: 13 in]
      }
    }
  }
